vi "Auto Setup.vi"(8 "error in":errorcluster) -> ()   [LabVIEW 2019]
uses:
  <vilib>/Rock Robotics/WPI/DriverStation/WPI_DriverStationRobotMode2.ctl
  9a55a8d7-5b3f-4802-bfcc-96ea82079109.vi
  Team Code/Robot Global Data.vi
  ed7fed8d-cbeb-403b-86f6-3c9ddeff16e0.vi
  <vilib>/Rock Robotics/Network Tables/NT Write String Array.vi
panel:
  in  "override":bool=TRUE
  out "error out":errorcluster
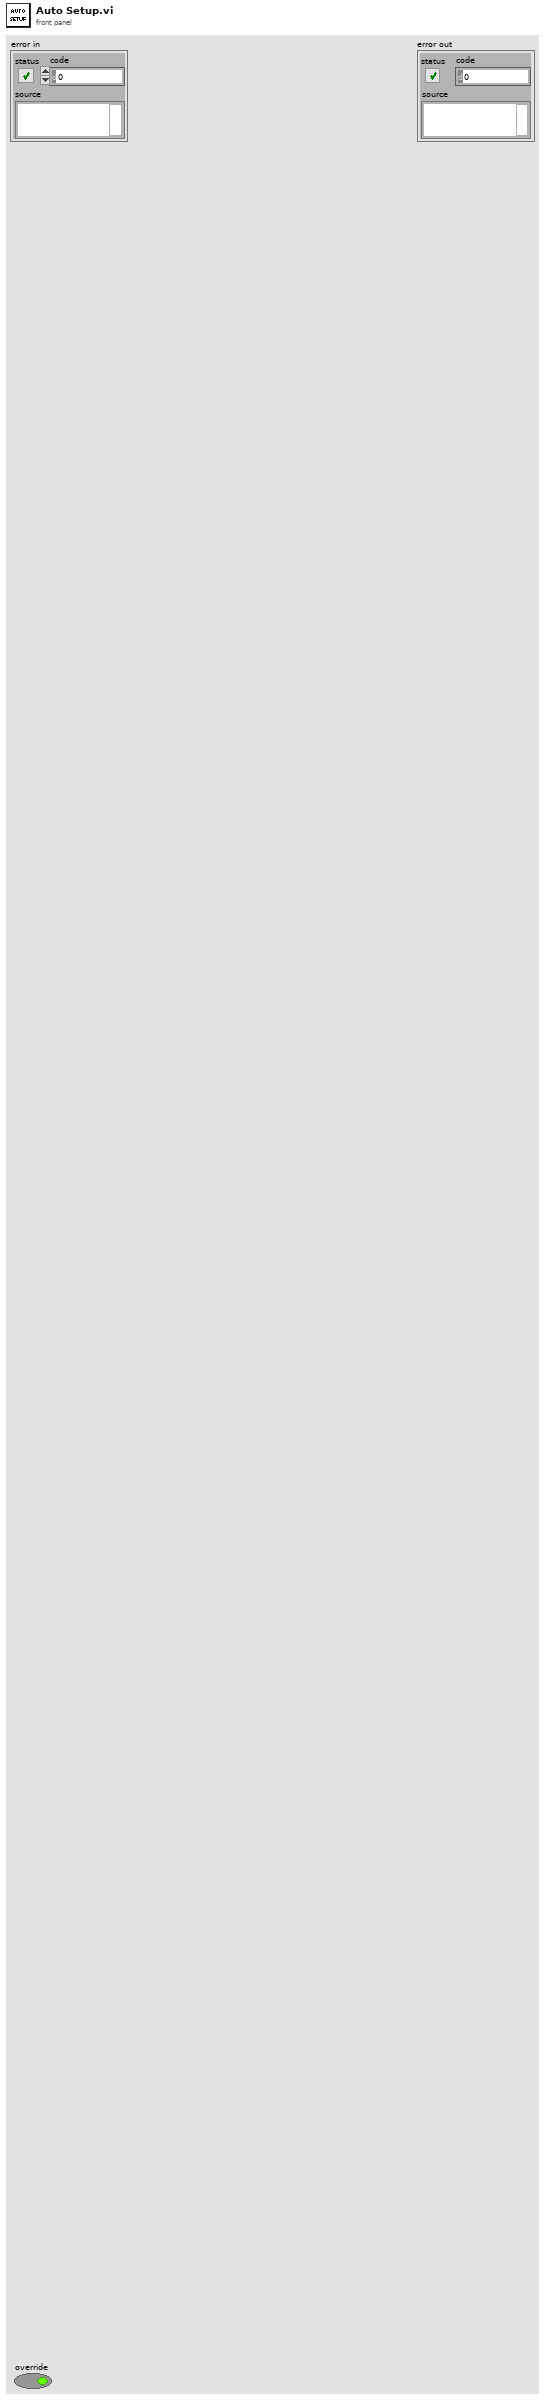
[diagram p1: front panel]
types:
  T1 = typedef "WPI_DriverStationRobotMode2.ctl" = enum16{"Autonomous Disabled", "Autonomous Enabled", "Teleop Disabled", "Teleop Enabled", "Disconnected", "Finish", "Test Disabled", "Test Enabled", "Emergency Stopped"}
  T2 = cluster{"Cluster":cluster{"Path Backwards":bool, "Robot Backwards":bool}, "Traj Vel Points":cluster{"V":dbl, "th":dbl}[], cluster{"Sample Period (s)":dbl, cluster{"Velocity (fps)":dbl, "Acceleration (fps^2)":dbl, "Jerk (fps^3)":dbl, dbl}, "Conditions":cluster{"vInitial (fps)":dbl, "vFinal (fps)":dbl}, "Angular Accelerations":cluster{"Angular \nAccelerations":dbl[], "Override Limits?":bool[]}}}
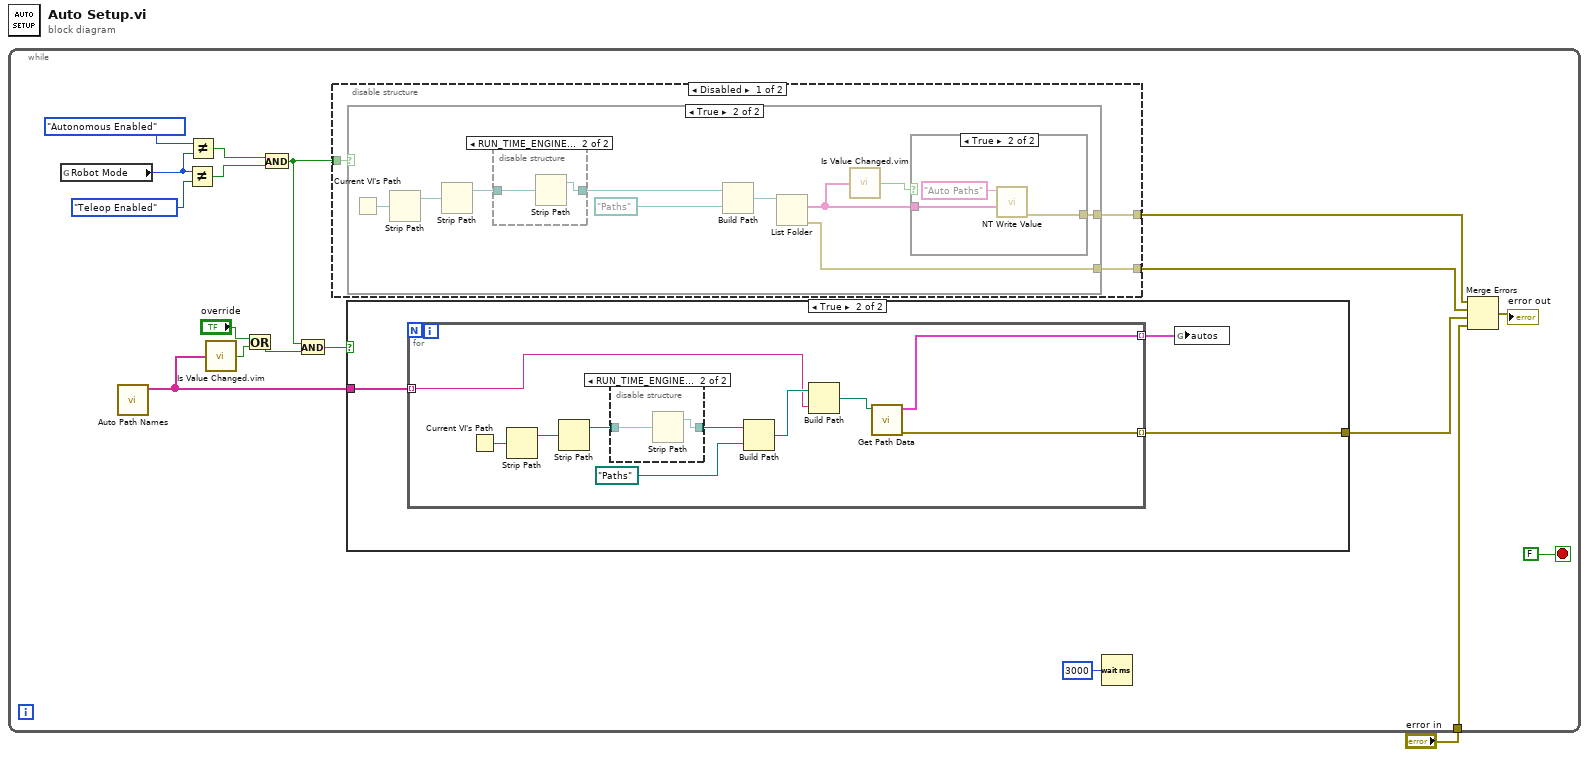
[diagram p0: block diagram]
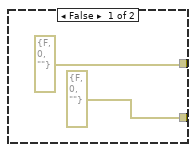
[diagram p2: hidden frame]
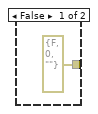
[diagram p3: hidden frame]
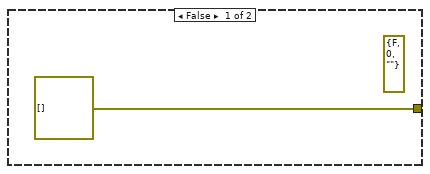
[diagram p6: hidden frame]
diagram:
  n1 = while {
    tunnel: "error in" -> [w10]
    stop <- FALSE stop-if-true
    n2 = global read "Robot Global Data.vi" "Robot Mode"() -> (w17:T1)
    n3 = call "Auto Path Names.vi"() -> ("Path Names"=w3:string[])  [unwired: 11 in]
    n4 = Not Equal?(x=w17, y=WPI_DriverStationRobotMode2."Teleop Enabled") -> (x != y?=w14:bool)
    n5 = Not Equal?(x=WPI_DriverStationRobotMode2."Autonomous Enabled", y=w17) -> (x != y?=w15:bool)
    n6 = call "Is Value Changed.vim"("value"=w3) -> ("changed or first call?"=w6:bool)
    n7 = Or(x="override", y=w6) -> (x .or. y?=w4:bool)
    n8 = And(x=w15, y=w14) -> (x .and. y?=w2:bool)
    n9 = And(x=w2, y=w4) -> (x .and. y?=w13:bool)
    n10 = disable-structure shown="Disabled" {
      disable-tunnel: [w22 _] -> w11
      disable-tunnel: [w21 _] -> w8
      disable-tunnel: w2 -> [w20 _]
      frame Disabled {
        n11 = case shown="True" w20 {
          tunnel: [errorcluster {"status"=FALSE, "code"=0, "source"=""} ("error out") w28] -> w22
          tunnel: [errorcluster {"status"=FALSE, "code"=0, "source"=""} ("error out") w27] -> w21
          frame False {
          }
          frame True {
            n12 = Current VI's Path() -> (path=w30:path)
            n13 = Strip Path(path=w30) -> (stripped path=w31:path)  [unwired: 1 out]
            n14 = Strip Path(path=w31) -> (stripped path=w33:path)  [unwired: 1 out]
            n15 = disable-structure shown="RUN_TIME_ENGINE==True, Default" {
              disable-tunnel: [w39 w40] -> w32
              disable-tunnel: w33 -> [w39 w41]
              frame condition #0 (active) {
              }
              frame condition #1 {
                n16 = Strip Path(path=w41) -> (stripped path=w40:path)  [unwired: 1 out]
              }
            }
            n17 = Build Path(base path=w32, name or relative path=path "Paths") -> (appended path=w34:path)
            n18 = List Folder(path=w34) -> (filenames=w26:string[], error out=w28:errorcluster)  [unwired: 3 in, 2 out]
            n19 = call "Is Value Changed.vim"("value"=w26) -> ("changed or first call?"=w25:bool)
            n20 = case shown="True" w25 {
              tunnel: w26 -> [_ w37]
              tunnel: [errorcluster {"status"=FALSE, "code"=0, "source"=""} ("error out") w36] -> w27
              frame False {
              }
              frame True {
                n21 = call-poly <vilib>:"NT Write Value.vi"("String Array"=w37, "Name"="Auto Paths") -> ("error out"=w36:errorcluster)  [unwired: 9 in]
              }
            }
          }
        }
      }
      frame Enabled {
      }
    }
    n22 = case shown="True" w13 {
      tunnel: w3 -> [_ w44]
      tunnel: [errorcluster[] [] w45] -> w12
      frame False {
        (unwired) errorcluster {"status"=FALSE, "code"=0, "source"=""} ("error out")
      }
      frame True {
        n23 = for {
          tunnel: w44 -> [w49] mode=indexing
          tunnel: [w47] -> w45 mode=indexing
          tunnel: [w46] -> w43 mode=indexing
          n24 = Current VI's Path() -> (path=w55:path)
          n25 = Strip Path(path=w55) -> (stripped path=w54:path)  [unwired: 1 out]
          n26 = Strip Path(path=w54) -> (stripped path=w52:path)  [unwired: 1 out]
          n27 = disable-structure shown="RUN_TIME_ENGINE==True, Default" {
            disable-tunnel: [w56 w57] -> w53
            disable-tunnel: w52 -> [w56 w58]
            frame condition #0 (active) {
            }
            frame condition #1 {
              n28 = Strip Path(path=w58) -> (stripped path=w57:path)  [unwired: 1 out]
            }
          }
          n29 = Build Path(base path=w53, name or relative path=path "Paths") -> (appended path=w50:path)
          n30 = Build Path(base path=w50, name or relative path=w49) -> (appended path=w48:path)
          n31 = call "Get Path Data.vi"("Path"=w48) -> ("error out"=w47:errorcluster, "Path stuff"=w46:T2)  [unwired: 9 in]
        }
        n32 = global write "Robot Global Data.vi" "autos"(w43) -> ()
      }
    }
    n33 = Wait (ms)(milliseconds to wait=u32 3000) -> ()  [unwired: 1 out]
    n34 = Merge Errors(w8, w11, w12, w10) -> (→"error out":errorcluster)
  }
